vi "Kinematics_Translation2d_RotateBy.vi"(9 "other Rotation":T1 {"SIN" format="%13.4f"; "COS" format="%13.4f"; "VALUE" format="%13.4f"}, 11 "In Translation":T2 {"Y" format="%14.3f"; "X" format="%14.3f"}) -> (3 "Out Translation":T2 {"Y" format="%14.3f"; "X" format="%14.3f"})   [LabVIEW 2020, in "Swerve_Odometry_SEN.lvlib"]
doc: "Applies a rotation to the translation in 2d space.\n\nThis multiplies the translation vector by a counterclockwise rotation matrix of the given angle.\n [x_new] [other.cos, -other.sin][x]\n [y_new] = [other.sin, other.cos][y]\n \nFor example, rotating a Translation2d of {2, 0} by 90 degrees will return a Translation2d of {0, 2}.\n\nParameters:\n - In Translation - This data structure\n - Other Rotation - The rotation to rotate the translation by. \n\nReturns:\n - Out Translation - The resulting Translation data structure"
uses:
  Swerve_Odometry_SEN.lvlib
  Cluster_TRANSLATION2D.ctl
  Cluster_ROTATION2D.ctl
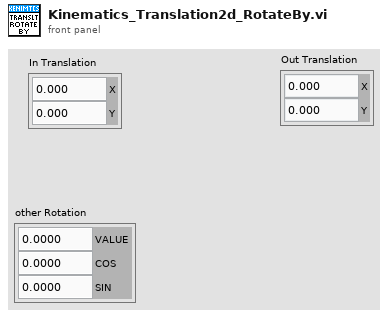
[diagram p1: front panel]
types:
  T1 = typedef "Swerve_Odometry_SEN.lvlib/Cluster_ROTATION2D.ctl" = cluster{"VALUE":dbl, "COS":dbl, "SIN":dbl}
  T2 = typedef "Swerve_Odometry_SEN.lvlib/Cluster_TRANSLATION2D.ctl" = cluster{"X":dbl, "Y":dbl}
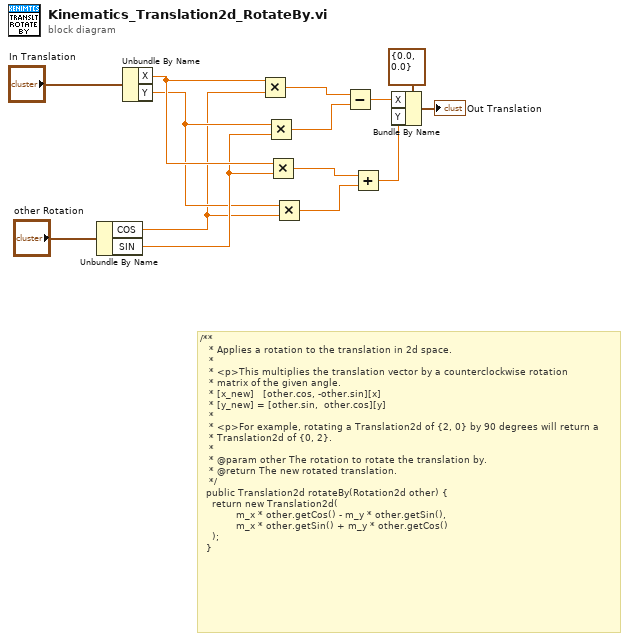
[diagram p0: block diagram]
diagram:
  # "/**\n   * Applies a rotation to the translation in 2d space.\n   *\n   * <p>This multiplies the translation vector by a counterclockwise rotation\n   * matrix of the given angle.\n   * [x_new]   [other.cos, -other.sin][x]\n   * [y_new] = [other.sin,  other.cos][y]\n   *\n   * <p>For example, rotating a Translation2d of {2, 0} by 90 degrees will return a\n   * Translation2d of {0, 2}.\n   *\n   * @param other The rotation to rotate the translation by.\n   * @return The new rotated translation.\n   */\n  public Translation2d rotateBy(Rotation2d other) {\n    return new Translation2d(\n            m_x * other.getCos() - m_y * other.getSin(),\n            m_x * other.getSin() + m_y * other.getCos()\n    );\n  }"
  n1 = Unbundle By Name("other Rotation") -> ("COS"=w5:dbl, "SIN"=w7:dbl)
  n2 = Unbundle By Name("In Translation") -> ("X"=w8:dbl, "Y"=w6:dbl)
  n3 = Multiply(x=w8, y=w5) -> (x*y=w12:dbl)
  n4 = Multiply(x=w6, y=w7) -> (x*y=w11:dbl)
  n5 = Multiply(x=w8, y=w7) -> (x*y=w10:dbl)
  n6 = Multiply(x=w6, y=w5) -> (x*y=w9:dbl)
  n7 = Subtract(x=w12, y=w11) -> (x-y=w1:dbl)
  n8 = Add(x=w10, y=w9) -> (x+y=w2:dbl)
  n9 = Bundle By Name(cluster=T2 {"X"=0.0, "Y"=0.0} ("TRANSLATION"), "X"=w1, "Y"=w2) -> (→"Out Translation":T2)
